vi "Multiple Camera Separator.vi"(11 "Detection Frame In":T1) -> (2 "Last Frame From Each Cam":T1[](array[typedef]), 3 "Last Frame":T1)   [LabVIEW 2016]
uses:
  SSL Detection Frame.ctl
  SSL Detection Robot.ctl
  SSL Detection Ball.ctl
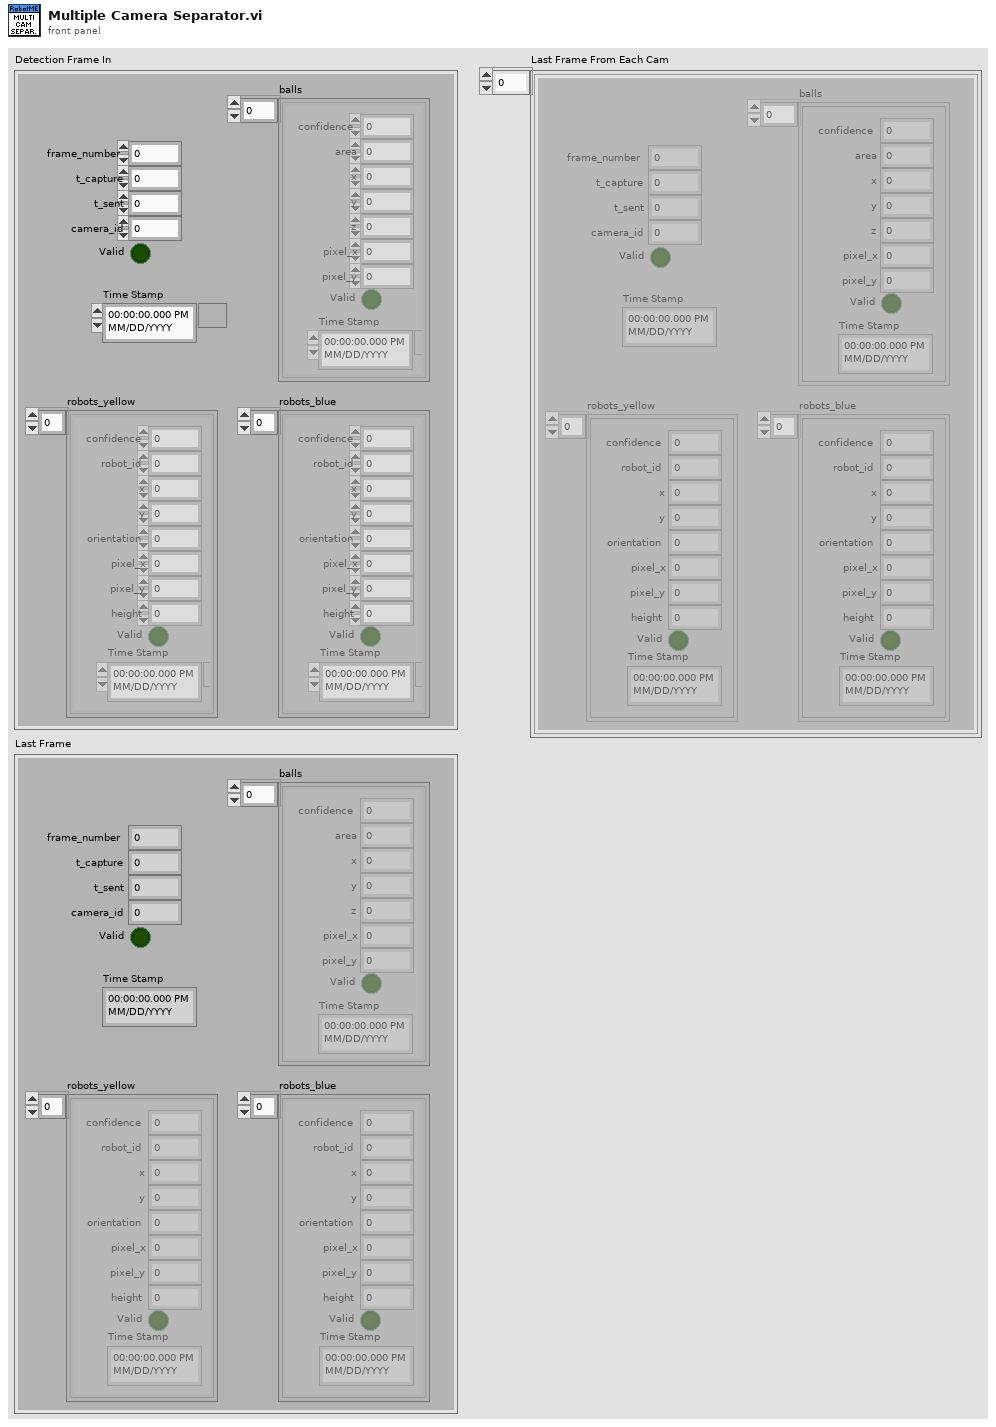
[diagram p1: front panel]
types:
  T1 = typedef "SSL Detection Frame.ctl" = cluster{"frame_number":u32, "t_capture":dbl, "t_sent":dbl, "camera_id":u32, "robots_yellow":T2[], "robots_blue":T2[], "balls":T3[], "Valid":bool, "Time Stamp":timestamp}
  T2 = typedef "SSL Detection Robot.ctl" = cluster{"x":dbl, "robot_id":u32, "confidence":sgl, "y":sgl, "orientation":sgl, "pixel_x":sgl, "pixel_y":sgl, "height":sgl, "Valid":bool, "Time Stamp":timestamp}
  T3 = typedef "SSL Detection Ball.ctl" = cluster{"x":sgl, "area":u32, "confidence":sgl, "y":sgl, "z":sgl, "pixel_x":sgl, "pixel_y":sgl, "Valid":bool, "Time Stamp":timestamp}
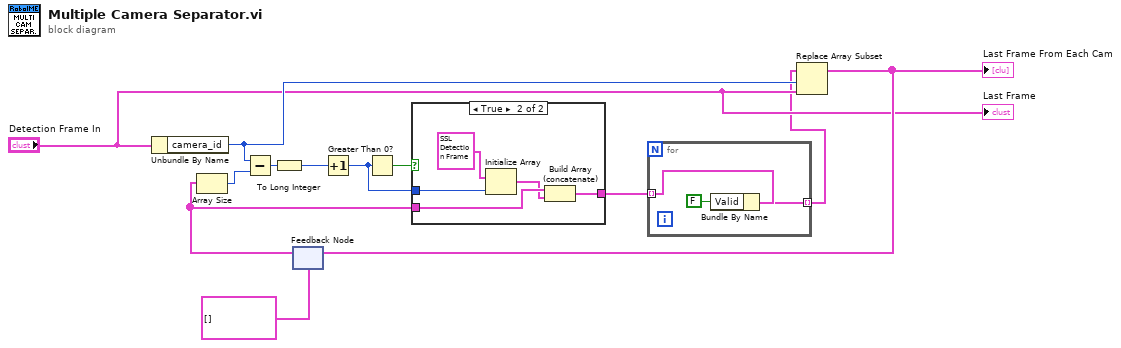
[diagram p0: block diagram]
diagram:
  n1 = Unbundle By Name("Detection Frame In") -> ("camera_id"=w9:u32)
  n2 = feedback #1(T1[] [] ("appended array")) -> (w10:T1[])
  n3 = Array Size(array=w10) -> (size(s)=w12:i32)
  n4 = Subtract(x=w9, y=w12) -> (x-y=w6:u32)
  n5 = To Long Integer(number=w6) -> (32bit integer=w4:i32)
  n6 = Increment(x=w4) -> (x+1=w3:i32)
  n7 = Greater Than 0?(x=w3) -> (x > 0?=w11:bool)
  n8 = case shown="True" w11 {
    tunnel: w3 -> [_ w17]
    tunnel: w10 -> [w13 w16]
    tunnel: [w13 w14] -> w2
    frame False {
    }
    frame True {
      n9 = Initialize Array(T1 {"frame_number"=0, "t_capture"=0.0, "t_sent"=0.0, "camera_id"=0, "robots_yellow"=[], "robots_blue"=[], "balls"=[], "Valid"=FALSE, "Time Stamp"=timestamp(0 s since 1904-01-01)} ("Detection Frame In 2"), w17) -> (w15:T1[])
      n10 = Build Array (concatenate)(w16, w15) -> (w14:T1[])
    }
  }
  n11 = for {
    tunnel: w2 -> [w21] mode=indexing
    tunnel: [w20] -> w1 mode=indexing
    n12 = Bundle By Name(cluster=w21, "Valid"=FALSE) -> (w20:T1)
  }
  n13 = Replace Array Subset(array=w1, new element="Detection Frame In", index=w9) -> (w8:T1[])
  "Last Frame From Each Cam" <- w8
  n14 = feedback-in #1(w8) -> ()
  "Last Frame" <- "Detection Frame In"
